vi "Route.vi"(8 "error in":errorcluster, 9 "Route To":string, 10 "Route From":string, 11 "34980A in":refnum<class "34980A.lvclass">) -> (0 "error out":errorcluster, 3 "34980A out":refnum<class "34980A.lvclass">)   [LabVIEW 2019, in "34980A.lvlib" / "34980A.lvclass"]
uses:
  Library/34980A.lvclass
  Library/34980A.lvclass/34980A.ctl
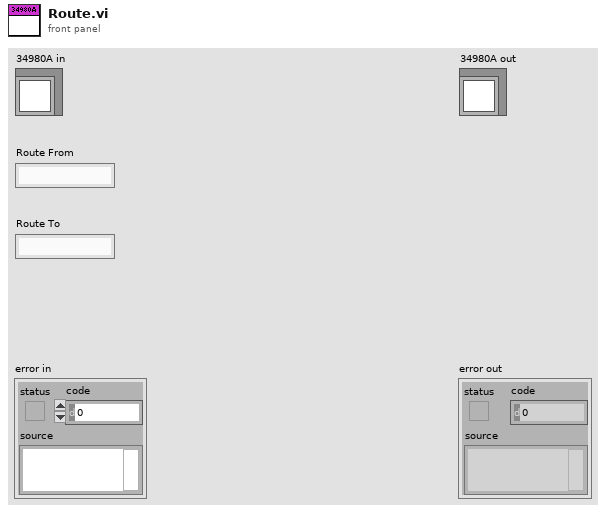
[diagram p1: front panel]
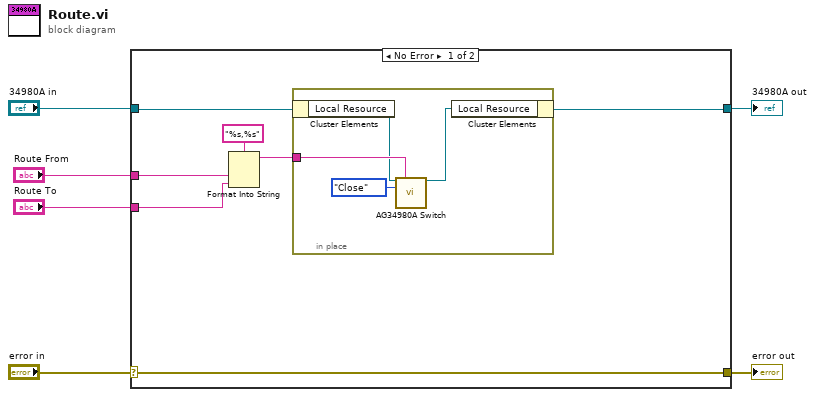
[diagram p0: block diagram]
diagram:
  n1 = case shown="No Error" "error in" {
    selector: "error in" -> [w13 w19]
    tunnel: [w13 w19] -> w5
    tunnel: [w7 w18] -> w3
    tunnel: "34980A in" -> [w8 w18]
    tunnel: "Route From" -> [w11 _]
    tunnel: "Route To" -> [w10 _]
    frame No Error {
      n2 = Format Into String(format string="%s,%s", w11, w10) -> (resulting string=w9:string)  [unwired: 2 in, 1 out]
      n3 = in-place {
        in-place-border: w9 -> [w17]
        n4 = in-place-cluster #1(w8) -> ("Local Resource"=w15:refnum<visa-resource-name>)
        n5 = call <instrlib>:"AG34980A Switch.vi"("VISA resource name"=w15, "Channel List"=w17, "Open/Close (0:Close)"=enum16{"Close", "Open"}."Close") -> ("VISA resource name out"=w14:refnum<visa-resource-name>)  [unwired: 10 in, 2 out]
        n6 = in-place-cluster #1("Local Resource"=w14) -> (w7:refnum<class "34980A.lvclass">)
      }
    }
    frame Error {
    }
  }
  "error out" <- w5
  "34980A out" <- w3
